vi "switch_load_extra.vi"(0 "Node":string, 1 "event time":string="045", 2 "Event type":string="CL", 3 "Fault type (phases)":string="BC") -> (7 "Event switches":string caption="Result")   [LabVIEW 2020]
panel:
  in  "Evento?":bool
  # "CHAVEAMENTO DE CARGA EXTRA\nPOR FASES (A, B, C ou combinações)"
  # "E se não encontrar a fase?\nNão vai fazer nada! simulação SEM evento"
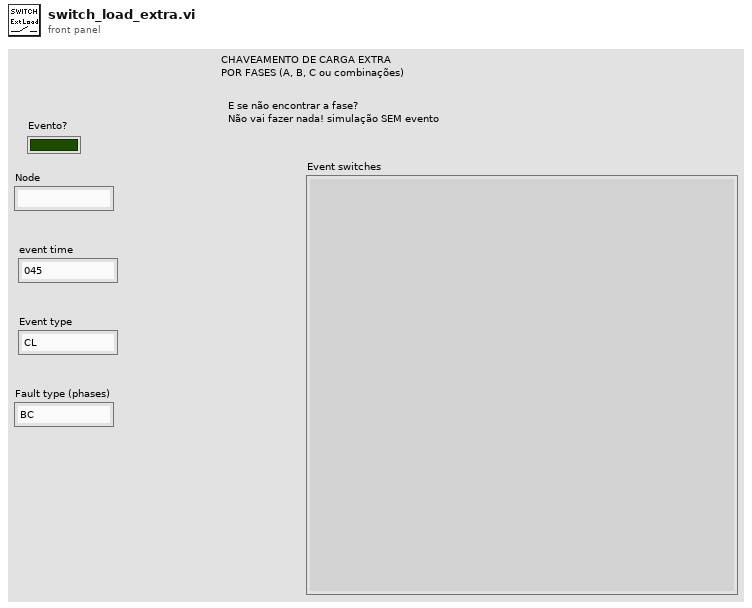
[diagram p1: front panel]
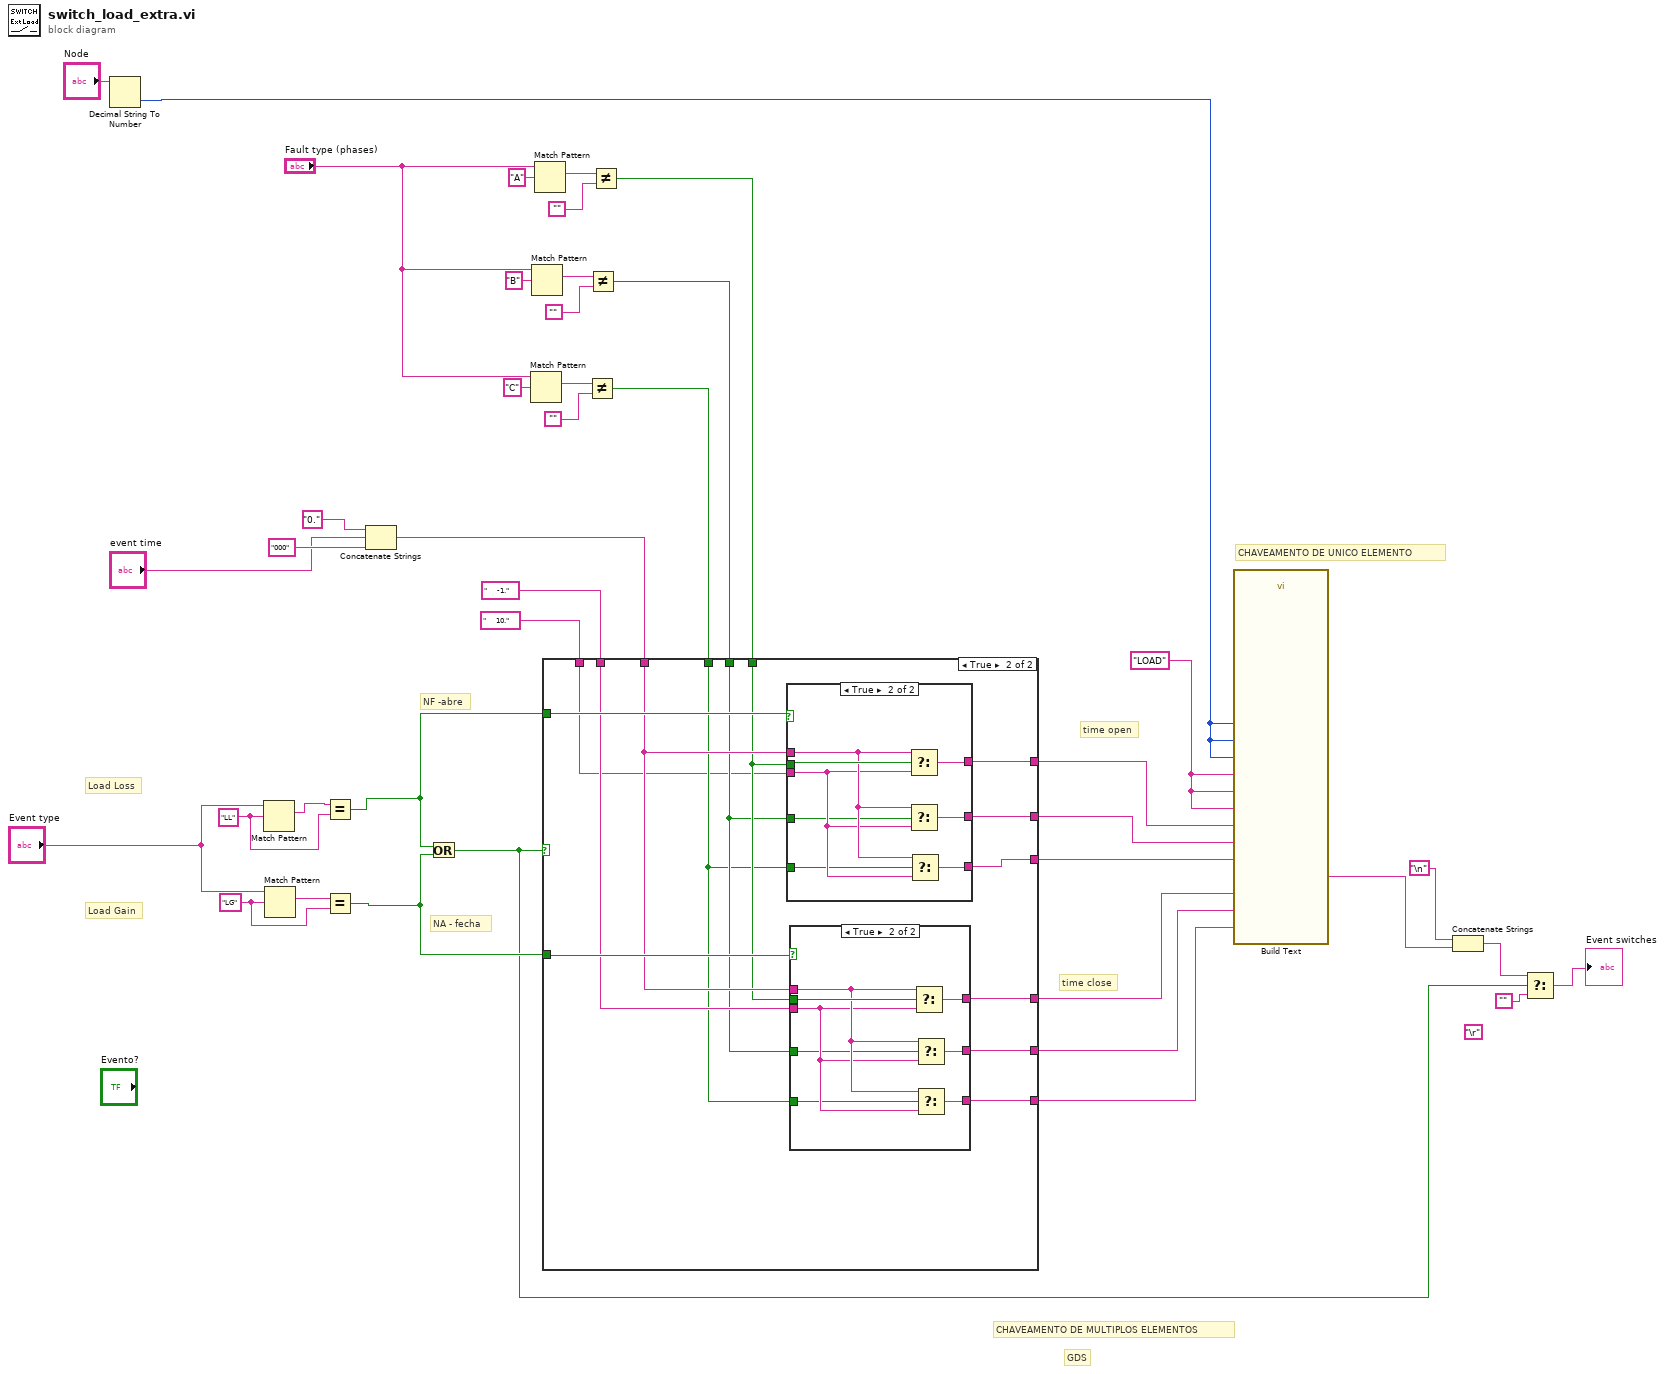
[diagram p0: block diagram]
diagram:
  w2 = "LOAD"
  (unwired) "\r"
  w36 = "LL" ("regular expression")
  w37 = "LG" ("regular expression")
  # "time close"
  # "time open"
  # "GDS"
  # "CHAVEAMENTO DE MULTIPLOS ELEMENTOS"
  # "CHAVEAMENTO DE UNICO ELEMENTO"
  # "NA - fecha"
  # "NF -abre"
  # "Load Gain"
  # "Load Loss"
  n1 = Decimal String To Number(string="Node") -> (number=w29:i32)  [unwired: 2 in, 1 out]
  n2 = Match Pattern(string="Event type", regular expression=w36) -> (match substring=w35:string)  [unwired: 1 in, 3 out]
  n3 = Match Pattern(string="Event type", regular expression=w37) -> (match substring=w39:string)  [unwired: 1 in, 3 out]
  n4 = Equal?(x=w35, y=w36) -> (x = y?=w28:bool)
  n5 = Equal?(x=w39, y=w37) -> (x = y?=w27:bool)
  n6 = Concatenate Strings("0." ("string"), "event time", "000" ("string")) -> (w30:string)
  n7 = Or(x=w28, y=w27) -> (x .or. y?=w26:bool)
  n8 = Match Pattern(string="Fault type (phases)", regular expression="C") -> (match substring=w16:string)  [unwired: 1 in, 3 out]
  n9 = Match Pattern(string="Fault type (phases)", regular expression="B") -> (match substring=w19:string)  [unwired: 1 in, 3 out]
  n10 = Match Pattern(string="Fault type (phases)", regular expression="A") -> (match substring=w22:string)  [unwired: 1 in, 3 out]
  n11 = Not Equal?(x=w16, y="") -> (x != y?=w9:bool)
  n12 = Not Equal?(x=w19, y="") -> (x != y?=w10:bool)
  n13 = Not Equal?(x=w22, y="") -> (x != y?=w11:bool)
  n14 = case shown="True" w26 {
    tunnel: w30 -> [_ w51]
    tunnel: "     -1." -> [w42 w52]
    tunnel: "     10." -> [w43 w44]
    tunnel: [w42 w50] -> w13
    tunnel: [w43 w57] -> w12
    tunnel: w27 -> [_ w53]
    tunnel: w28 -> [_ w56]
    tunnel: w11 -> [_ w49]
    tunnel: [w43 w55] -> w7
    tunnel: [w43 w54] -> w8
    tunnel: w10 -> [_ w48]
    tunnel: w9 -> [_ w47]
    tunnel: [w42 w46] -> w6
    tunnel: [w42 w45] -> w5
    frame False {
    }
    frame True {
      n15 = case shown="True" w56 {
        tunnel: [w67 w75] -> w57
        tunnel: w51 -> [_ w72]
        tunnel: w44 -> [w67 w71]
        tunnel: w49 -> [_ w74]
        tunnel: [w67 w73] -> w54
        tunnel: [w67 w70] -> w55
        tunnel: w48 -> [_ w69]
        tunnel: w47 -> [_ w68]
        frame False {
        }
        frame True {
          n16 = Select(t=w72, s=w74, f=w71) -> (s? t:f=w75:string)
          n17 = Select(t=w72, s=w69, f=w71) -> (s? t:f=w73:string)
          n18 = Select(t=w72, s=w68, f=w71) -> (s? t:f=w70:string)
        }
      }
      n19 = case shown="True" w53 {
        tunnel: w52 -> [w58 w63]
        tunnel: w51 -> [_ w64]
        tunnel: [w58 w66] -> w50
        tunnel: w49 -> [_ w65]
        tunnel: w48 -> [_ w62]
        tunnel: w47 -> [_ w61]
        tunnel: [w58 w60] -> w46
        tunnel: [w58 w59] -> w45
        frame False {
        }
        frame True {
          n20 = Select(t=w64, s=w65, f=w63) -> (s? t:f=w66:string)
          n21 = Select(t=w64, s=w62, f=w63) -> (s? t:f=w60:string)
          n22 = Select(t=w64, s=w61, f=w63) -> (s? t:f=w59:string)
        }
      }
    }
  }
  n23 = call "Build Text"("inA"=w29, "inA_2"=w2, "time_close_A"=w13, "time_open_A"=w12, "inB"=w29, "inB_2"=w2, "time_close_B"=w6, "time_open_B"=w8, "inC"=w29, "inC_2"=w2, "time_close_C"=w5, "time_open_C"=w7) -> ("Result"=w3:string)  [unwired: 14 in, 1 out]
  n24 = Concatenate Strings("\n", w3) -> (w24:string)
  n25 = Select(t=w24, s=w26, f="") -> (s? t:f=→"Event switches":string)
